vi "TSC Material UI Surface Level--constant.vi"() -> (2 "UI surface levels":string[](array[string]))   [LabVIEW 2021]
doc: "This VI defines the constant value for the UI Surface Levels that are shown in the right click menu and are used in color application.\n\n\n<b>Code Developed By:</b>\nTechnology Service Corporation\n1983 S Liberty Drive\nBloomington, IN 47403\nwww.tsc.com/atcs\n\nDeveloper:\nDaniel Coons"
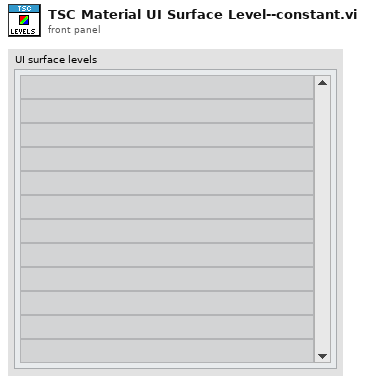
[diagram p1: front panel]
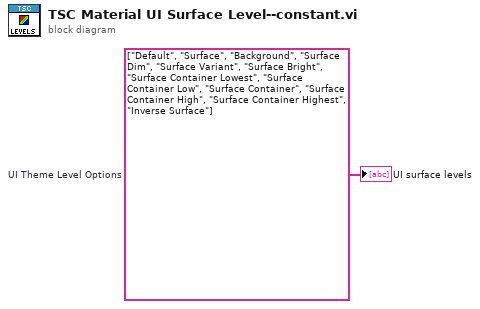
[diagram p0: block diagram]
diagram:
  w1 = string[] ["Default", "Surface", "Background", "Surface Dim", "Surface Variant", "Surface Bright", "Surface Container Lowest", "Surface Container Low", "Surface Container", "Surface Container High", "Surface Container Highest", "Inverse Surface"]  # UI Theme Level Options
  "UI surface levels" <- w1
